vi "dataAcquisition.vi"() -> ()   [LabVIEW 2018]
uses:
  PCI8552B_32.DLL
panel:
  out "波形图":dbl[][](graph)
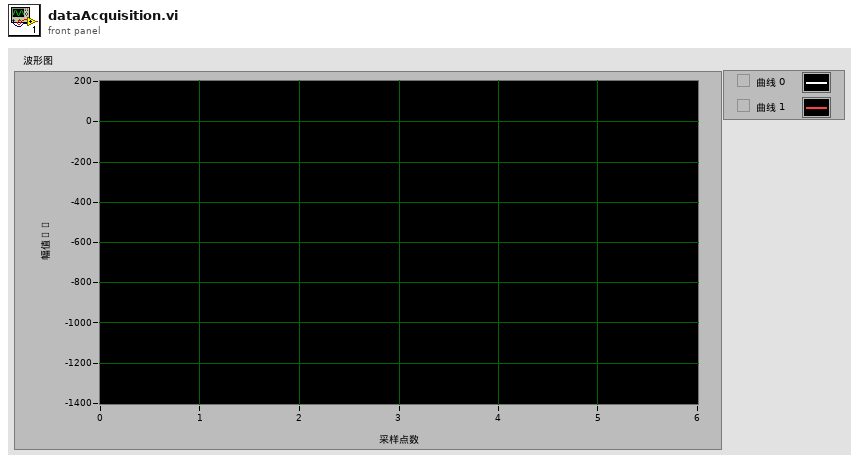
[diagram p1: front panel]
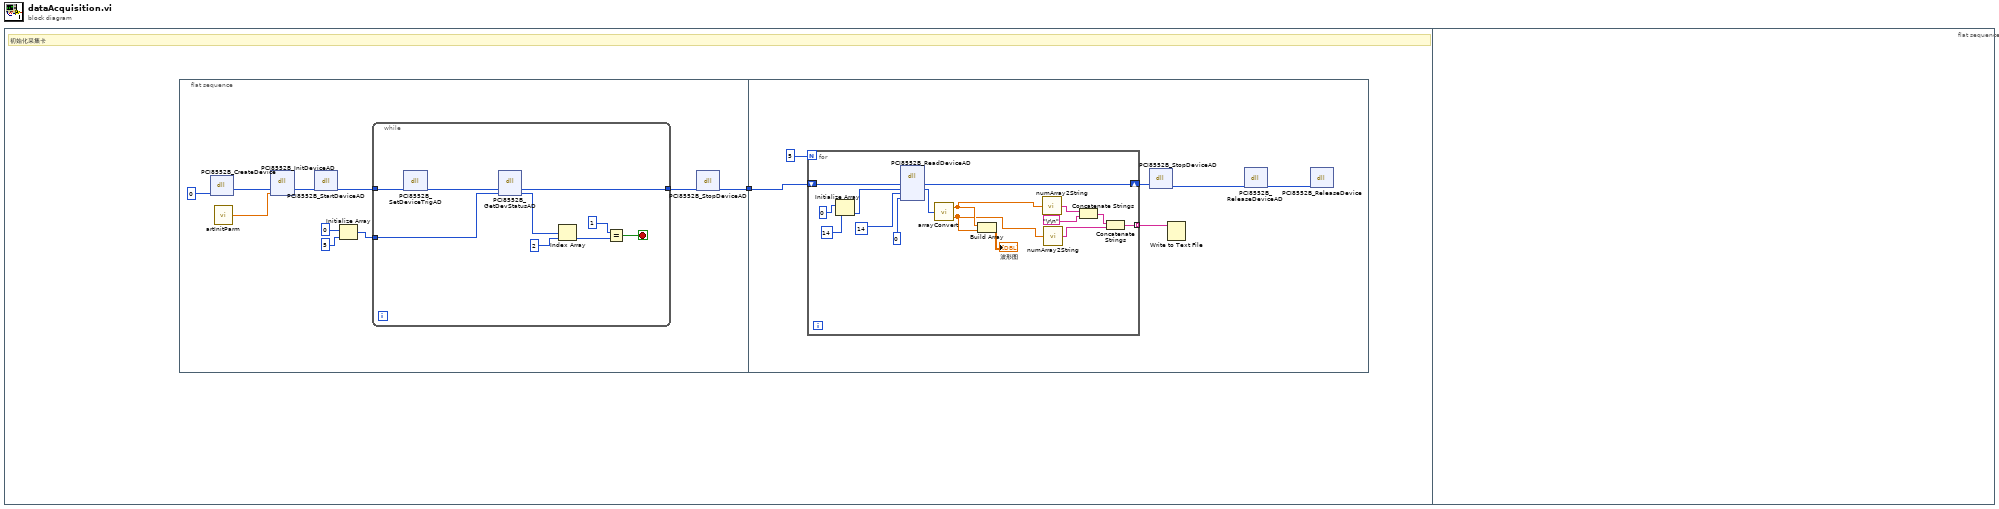
[diagram p0: block diagram]
diagram:
  n1 = flat-sequence {
    frame #0 {
      # "初始化采集卡"
      n2 = flat-sequence {
        tunnel: [w7] -> w1
        tunnel: w1 -> [w22]
        frame #0 {
          n3 = dll-call lib="PCI8552B_32" fn="PCI8552B_CreateDevice" label="CreateDevice"("DeviceLgcID"=0) -> ("返回类型"=w4:i32)  [unwired: 4 in, 2 out]
          n4 = call "artInitParm.vi"() -> ("初始化参数"=w6:dbl[])
          n5 = dll-call lib="PCI8552B_32.DLL" fn="PCI8552B_InitDeviceAD" label="InitDeviceAD"("hDevice"=w4, "pADPara"=w6) -> ("hDevice"=w5:i32)  [unwired: 5 in, 2 out]
          n6 = dll-call lib="PCI8552B_32.DLL" fn="PCI8552B_StartDeviceAD" label="StartDeviceAD"("hDevice"=w5) -> ("hDevice"=w2:i32)  [unwired: 4 in, 2 out]
          n7 = Initialize Array(0, 5) -> (w11:i32[])
          n8 = while {
            tunnel: w2 -> [w15]
            tunnel: w11 -> [w20]
            tunnel: [w13] -> w8
            stop <- w12 stop-if-true
            n9 = dll-call lib="PCI8552B_32.DLL" fn="PCI8552B_SetDeviceTrigAD" label="SetDeviceTrigAD"("hDevice"=w15) -> ("hDevice"=w14:i32)  [unwired: 4 in, 2 out]
            n10 = dll-call lib="PCI8552B_32.DLL" fn="PCI8552B_GetDevStatusAD" label="GetDevStatusAD"("hDevice"=w14, "ADStatus"=w20) -> ("hDevice"=w13:i32, "ADStatus"=w16:i32[])  [unwired: 4 in, 2 out]
            n11 = Index Array(array=w16, index=2) -> (element=w18:i32)
            n12 = Equal?(x=1, y=w18) -> (x = y?=w12:bool)
          }
          n13 = dll-call lib="PCI8552B_32.DLL" fn="PCI8552B_StopDeviceAD" label="StopDeviceAD"("hDevice"=w8) -> ("hDevice"=w7:i32)  [unwired: 4 in, 2 out]
        }
        frame #1 {
          n14 = for {
            N: u16 5 ("y") -> [_]
            shift-right: [w40] -> w26
            shift-left: w22 -> [w41]
            tunnel: [w31] -> w21 mode=indexing
            n15 = Initialize Array(u16 0 ("y"), 14 ("y")) -> (w27:u16[])
            n16 = dll-call lib="PCI8552B_32.DLL" fn="PCI8552B_ReadDeviceAD" label="ReadDeviceAD"("hDevice"=w41, "pADBuffer"=w27, "nReadSizeWords"=14 ("y"), "nRetSizeWords"=u16 0 ("y")) -> ("hDevice"=w40:i32, "pADBuffer"=w39:u16[])  [unwired: 6 in, 2 out]
            n17 = call "arrayConvert.vi"("输入数组"=w39) -> ("通道0输出"=w36:dbl[], "通道1输出"=w35:dbl[])
            n18 = Build Array ("创建数组")(w36, w35) -> (→"波形图":dbl[][])
            n19 = call "numArray2String.vi"("输入数组"=w36) -> ("输出字符串"=w34:string)
            n20 = call "numArray2String.vi"("输入数组"=w35) -> ("输出字符串"=w30:string)
            n21 = Concatenate Strings(w34, "\r\n") -> (w32:string)
            n22 = Concatenate Strings(w32, w30) -> (w31:string)
          }
          n23 = dll-call lib="PCI8552B_32.DLL" fn="PCI8552B_StopDeviceAD" label="StopDeviceAD"("hDevice"=w26) -> ("hDevice"=w24:i32)  [unwired: 4 in, 2 out]
          n24 = Write to Text File(text=w21) -> ()  [unwired: 3 in, 3 out]
          n25 = dll-call lib="PCI8552B_32.DLL" fn="PCI8552B_ReleaseDeviceAD" label="ReleaseDeviceAD"("hDevice"=w24) -> ("hDevice"=w25:i32)  [unwired: 4 in, 2 out]
          n26 = dll-call lib="PCI8552B_32.DLL" fn="PCI8552B_ReleaseDevice" label="ReleaseDevice"("hDevice"=w25) -> ()  [unwired: 5 in, 2 out]
        }
      }
    }
    frame #1 {
    }
  }
